vi "Do.vi"(8 "error in":errorcluster, 10 "Actor in":refnum<class "Actor.lvclass">, 11 "Set Voffset MSG":refnum<class "Set Voffset MSG.lvclass">) -> (0 "error out":errorcluster, 2 "Actor out":refnum<class "Actor.lvclass">)   [LabVIEW 2014, in "ePAS Library.lvlib" / "Set Voffset MSG.lvclass"]
doc: "(<B>Filename</B>: Actor Framework.lvlib:Message.lvclass:Do.vi)\n\nDefines what a message does when it is received by an actor. Generally, a message instructs an actor to invoke one of its methods. By default, this method does nothing. A child class must override it to define behavior. Create a child class by using the Actor Framework Message Maker dialog box."
uses:
  Set Voffset MSG.lvclass
  <vilib>/ActorFramework/Actor/Actor.lvclass
  Set Voffset MSG.lvclass/Set Voffset MSG.ctl
  Instr Actor.lvclass
  PAS/Commands/Change Laser Voffset/Change Laser Voffset.lvclass
  PAS/Commands/Change Laser Voffset/Change Laser Voffset.lvclass/Change Laser Voffset.ctl
  PAS/Commands/Change Laser Voffset/Write Voffset.vi
  reusable/Command/Command.lvclass
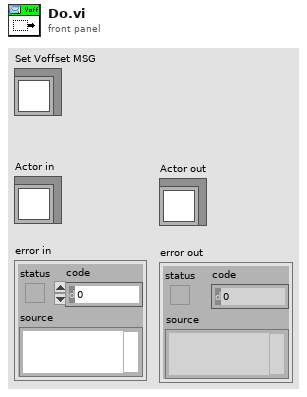
[diagram p1: front panel]
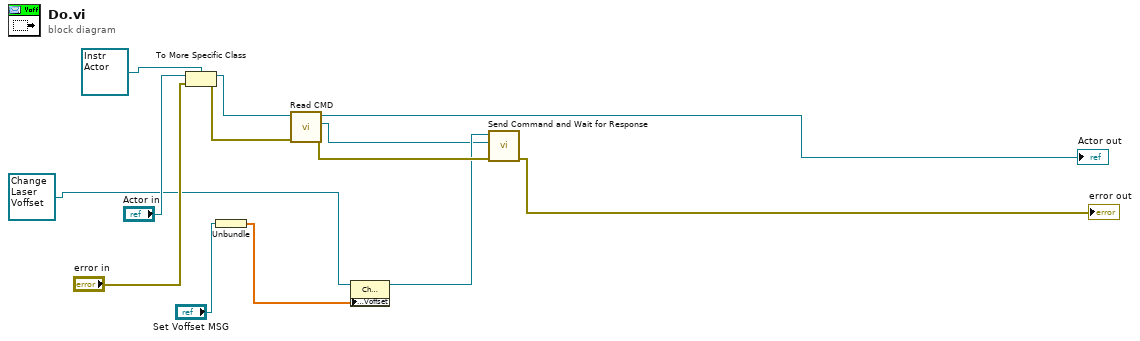
[diagram p0: block diagram]
diagram:
  n1 = To More Specific Class(target class=refnum<class "Instr Actor.lvclass"> refnum ("Instrument Lib:Instr"), reference="Actor in", error in="error in") -> (specific class reference=w11:refnum<class "Instr Actor.lvclass">, error out=w10:errorcluster)
  n2 = Unbundle("Set Voffset MSG") -> (w1:sgl[])
  n3 = call "Read CMD.vi"("error in (no error)"=w10, "Instr Actor in"=w11) -> ("error out"=w7:errorcluster, "CMD"=w4:refnum<queue>, "Instr Actor out"=→"Actor out":refnum<class "Instr Actor.lvclass">)  [unwired: 7 in]
  n4 = property class="Change Laser Voffset.lvclass"(reference=refnum<class "Change Laser Voffset.lvclass"> refnum ("Change Laser Voffset.lvclass"), "Accessors:Voffset"=w1) -> (reference out=w5:refnum<class "Change Laser Voffset.lvclass">)  [unwired: 1 in, 1 out]
  n5 = call "Send Command and Wait for Response.vi"("error in"=w7, "cmd queue"=w4, "CMD in"=w5) -> ("error out"=→"error out":errorcluster)  [unwired: 6 in, 2 out]
